vi "Match Pattern vs Match Reg Pattern.vi"() -> ()   [LabVIEW 2020]
uses:
  <vilib>/regexp/Match Regular Expression.xnode
panel:
  out "unit (ms) 2":dbl[](graph)
  out "inside 2":i32
  out "outside 2":i32
  out "inside":i32
  out "outside":i32
  out "unit (ms)":dbl[][](graph)
  out "Boolean 2":bool
  out "Boolean":bool
  out "whole match":string
  out "string":string
  # "Match Pattern vs Match Reg Pattern.vi"
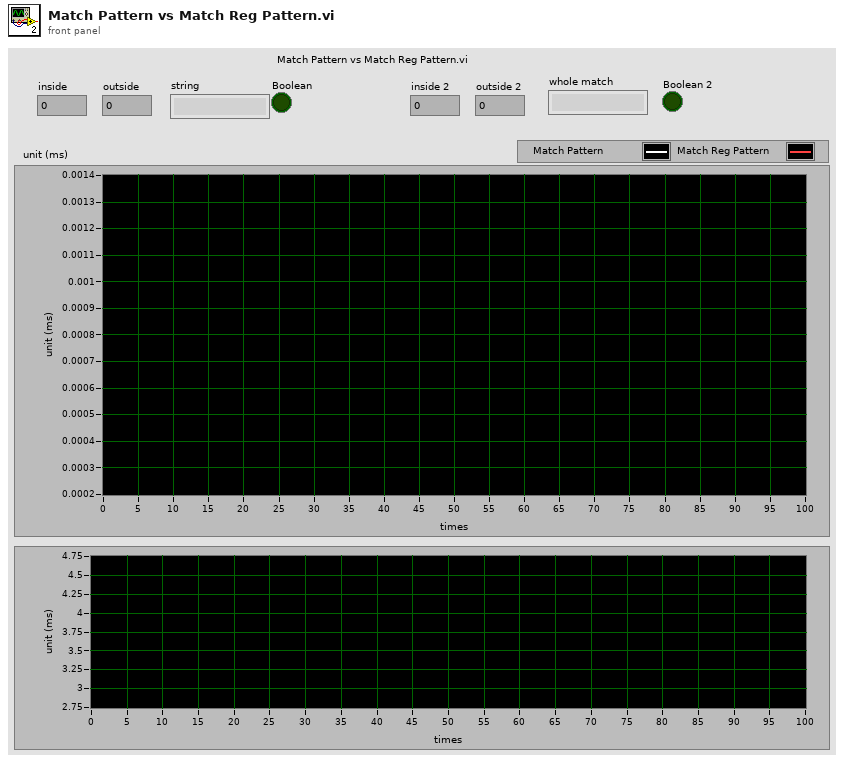
[diagram p1: front panel]
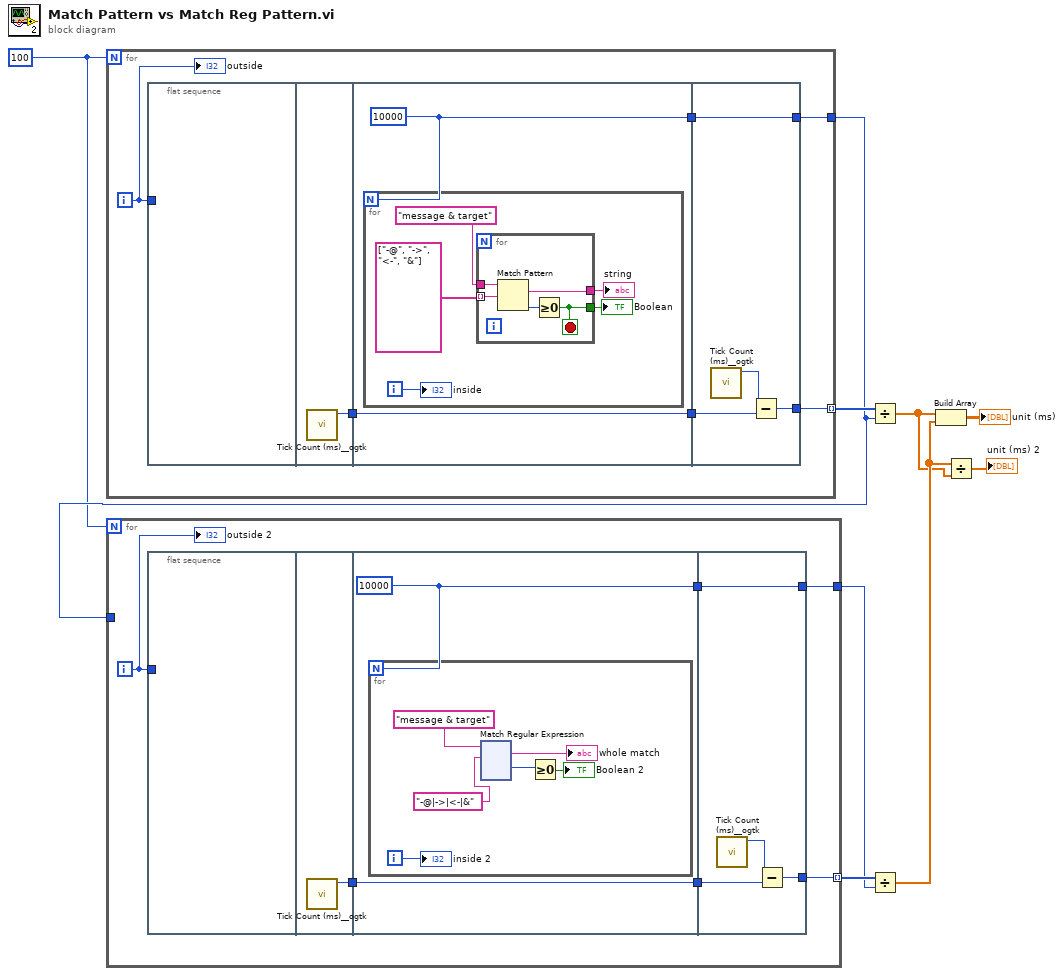
[diagram p0: block diagram]
diagram:
  w4 = 100
  n1 = for {
    N: w4 -> [_]
    tunnel: [w13] -> w9 mode=indexing
    tunnel: [w12] -> w5
    i -> [w10]
    n2 = flat-sequence {
      tunnel: w10 -> [_]
      tunnel: [w16] -> w15
      tunnel: w15 -> [w18]
      tunnel: [w18] -> w14
      tunnel: [w17] -> w11
      tunnel: w14 -> [w31]
      tunnel: [w30] -> w13
      tunnel: [w29] -> w12
      tunnel: w11 -> [w29]
      frame #0 {
      }
      frame #1 {
        n3 = call <userlib>:"Tick Count (ms)__ogtk.vi"() -> ("millisecond timer value"=w16:u32)  [unwired: 10 in, 1 out]
      }
      frame #2 {
        w17 = 10000
        n4 = for {
          N: w17 -> [_]
          i -> [w23]
          n5 = for {
            tunnel: string[] ["-@", "->", "<-", "&"] -> [w28] mode=indexing
            tunnel: [w26] -> w21
            tunnel: [w25] -> w22
            tunnel: "message & target" ("string") -> [w24]
            stop <- w25 stop-if-true
            n6 = Match Pattern(string=w24, regular expression=w28) -> (match substring=w26:string, offset past match=w27:i32)  [unwired: 1 in, 2 out]
            n7 = Greater Or Equal To 0?(x=w27) -> (x >= 0?=w25:bool)
          }
          "string" <- w21
          "Boolean" <- w22
          "inside" <- w23
        }
      }
      frame #3 {
        n8 = call <userlib>:"Tick Count (ms)__ogtk.vi"() -> ("millisecond timer value"=w32:u32)  [unwired: 10 in, 1 out]
        n9 = Subtract(x=w32, y=w31) -> (x-y=w30:u32)
      }
    }
    "outside" <- w10
  }
  n10 = for {
    N: w4 -> [_]
    tunnel: [w36] -> w7 mode=indexing
    tunnel: [w35] -> w6
    tunnel: w5 -> [_]
    i -> [w33]
    n11 = flat-sequence {
      tunnel: w33 -> [_]
      tunnel: [w39] -> w38
      tunnel: w38 -> [w41]
      tunnel: [w41] -> w37
      tunnel: [w40] -> w34
      tunnel: w37 -> [w164]
      tunnel: [w163] -> w36
      tunnel: [w162] -> w35
      tunnel: w34 -> [w162]
      frame #0 {
      }
      frame #1 {
        n12 = call <userlib>:"Tick Count (ms)__ogtk.vi"() -> ("millisecond timer value"=w39:u32)  [unwired: 10 in, 1 out]
      }
      frame #2 {
        w40 = 10000
        n13 = for {
          N: w40 -> [_]
          i -> [w47]
          n14 = xnode "Match Regular Expression"("input string"="message & target", "regular expression"="-@|->|<-|&") -> ("whole match"=→"whole match":string, "offset past match"=w45:i32)  [unwired: 4 in, 3 out]
          n15 = Greater Or Equal To 0?(x=w45) -> (x >= 0?=→"Boolean 2":bool)
          "inside 2" <- w47
        }
      }
      frame #3 {
        n16 = call <userlib>:"Tick Count (ms)__ogtk.vi"() -> ("millisecond timer value"=w165:u32)  [unwired: 10 in, 1 out]
        n17 = Subtract(x=w165, y=w164) -> (x-y=w163:u32)
      }
    }
    "outside 2" <- w33
  }
  n18 = Divide(x=w9, y=w5) -> (x/y=w2:dbl[])
  n19 = Divide(x=w7, y=w6) -> (x/y=w3:dbl[])
  n20 = Build Array(w2, w3) -> (→"unit (ms)":dbl[][])
  n21 = Divide(x=w3, y=w2) -> (x/y=→"unit (ms) 2":dbl[])
